vi "SDCP - Read parameter file.vi"(2 "error in (no error)":errorcluster, 3 "Parameter file path":path) -> (0 "error out":errorcluster, 1 "Parameter descriptors":T1[](array[typedef]))   [LabVIEW 2020]
uses:
  Typedefs/SDCP - SMF parameter descriptors.ctl
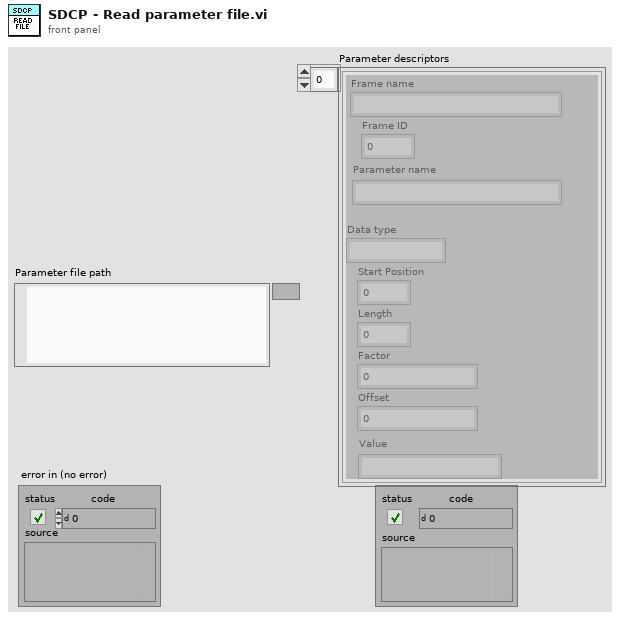
[diagram p1: front panel]
types:
  T1 = typedef "SDCP - SMF parameter descriptors.ctl" = cluster{"Frame name":string, "Frame ID":i32, "Data type":string, "Start Position":i32, "Length":i32, "Factor":dbl, "Offset":dbl, "Parameter name":string, "Value":string}
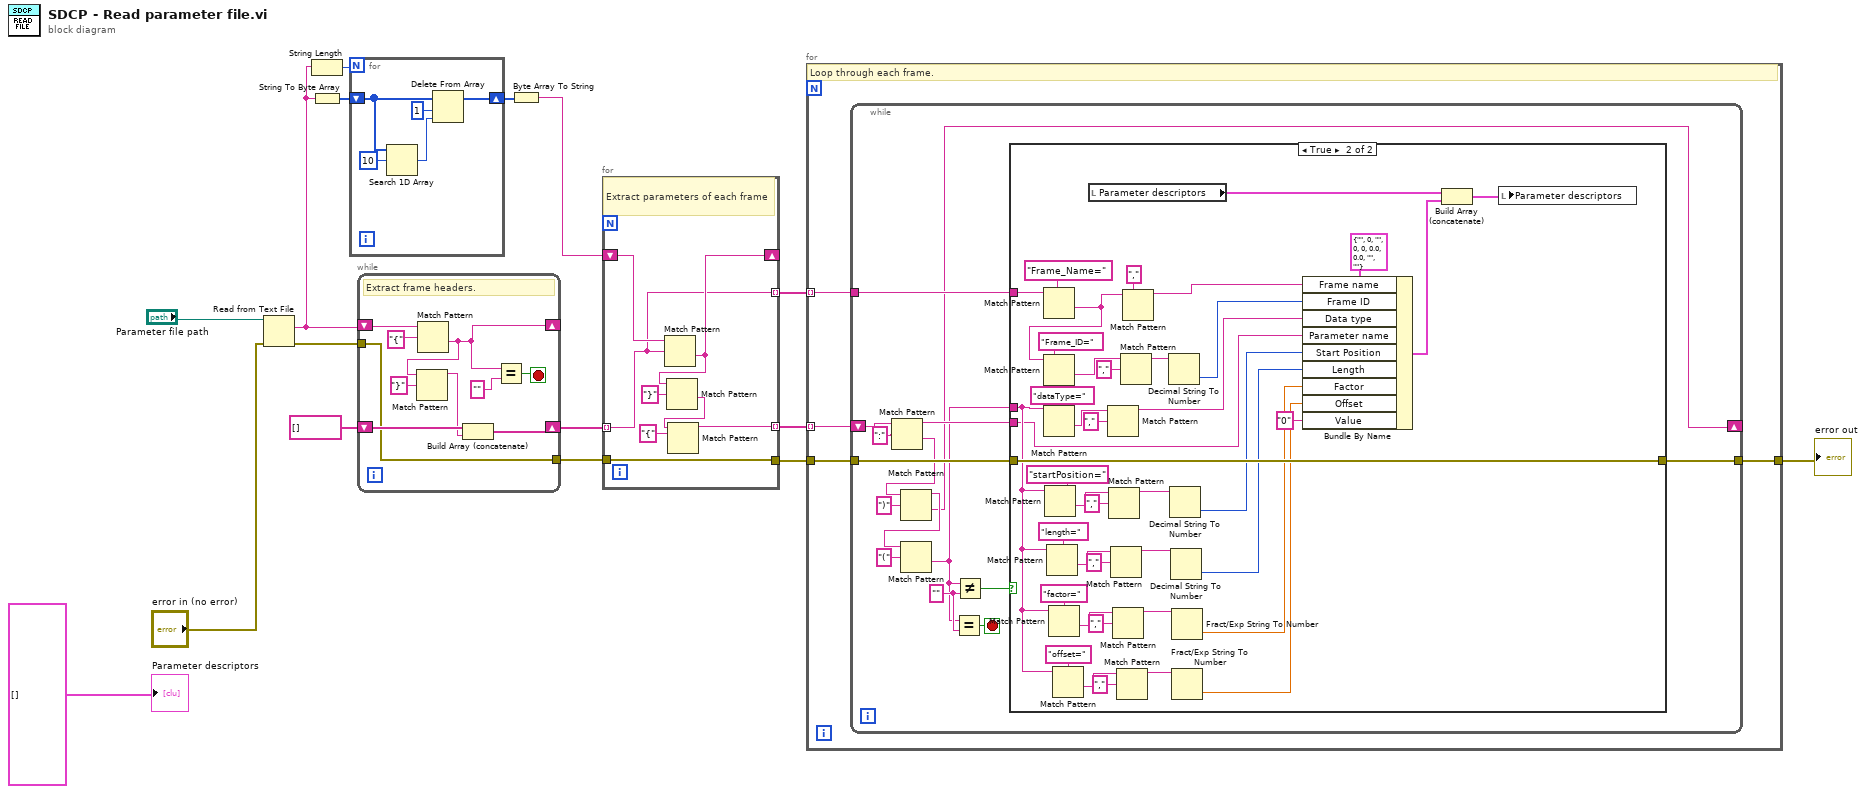
[diagram p0: block diagram]
diagram:
  n1 = Read from Text File(file (use dialog)="Parameter file path", error in="error in (no error)") -> (text=w3:string, error out=w14:errorcluster)  [unwired: 2 in, 2 out]
  n2 = String Length(string=w3) -> (length=w4:i32)
  n3 = String To Byte Array(string=w3) -> (unsigned byte array=w7:u8[])
  n4 = for {
    N: w4 -> [_]
    shift-right: [w21] -> w6
    shift-left: w7 -> [w20]
    n5 = Search 1D Array(1D array=w20, element=u8 10) -> (index of element=w17:i32)  [unwired: 1 in]
    n6 = Delete From Array(array=w20, length=1, index=w17) -> (array with subset deleted=w21:u8[])  [unwired: 1 out]
  }
  n7 = while {
    tunnel: w14 -> [w22]
    shift-right: [w25] -> _
    shift-left: w3 -> [w31]
    shift-right: [w26] -> w12
    shift-left: string[] [] -> [w28]
    tunnel: [w22] -> w11
    stop <- w24 stop-if-true
    # "Extract frame headers."
    n8 = Match Pattern(string=w31, regular expression="{") -> (after substring=w25:string)  [unwired: 1 in, 3 out]
    n9 = Match Pattern(string=w25, regular expression="}") -> (before substring=w27:string)  [unwired: 1 in, 3 out]
    n10 = Build Array (concatenate)(w28, w27) -> (w26:string[])
    n11 = Equal?(x=w25, y="") -> (x = y?=w24:bool)
  }
  n12 = Byte Array To String(unsigned byte array=w6) -> (string=w5:string)
  n13 = for {
    tunnel: w12 -> [w33] mode=indexing
    tunnel: w11 -> [w32]
    shift-right: [w35] -> _
    shift-left: w5 -> [w39]
    tunnel: [w34] -> w9 mode=indexing
    tunnel: [w33] -> w8 mode=indexing
    tunnel: [w32] -> w10
    # "Extract parameters of each frame"
    n14 = Match Pattern(string=w39, regular expression=w33) -> (after substring=w35:string)  [unwired: 1 in, 3 out]
    n15 = Match Pattern(string=w35, regular expression="}") -> (after substring=w38:string)  [unwired: 1 in, 3 out]
    n16 = Match Pattern(string=w38, regular expression="{") -> (before substring=w34:string)  [unwired: 1 in, 3 out]
  }
  n17 = for {
    tunnel: w10 -> [w41]
    tunnel: w9 -> [w42] mode=indexing
    tunnel: w8 -> [w43] mode=indexing
    tunnel: [w40] -> w1
    # "Loop through each frame."
    n18 = while {
      tunnel: w43 -> [w50]
      tunnel: w41 -> [w52]
      tunnel: [w51] -> w40
      shift-right: [w44] -> _
      shift-left: w42 -> [w49]
      stop <- w53 stop-if-true
      w54 = "" ("y")
      n19 = Match Pattern(string=w49, regular expression=":") -> (before substring=w46:string, after substring=w47:string)  [unwired: 1 in, 2 out]
      n20 = Match Pattern(string=w47, regular expression=")") -> (before substring=w57:string, after substring=w44:string)  [unwired: 1 in, 2 out]
      n21 = Match Pattern(string=w57, regular expression="(") -> (after substring=w45:string)  [unwired: 1 in, 3 out]
      n22 = Equal?(x=w45, y=w54) -> (x = y?=w53:bool)
      n23 = Not Equal?(x=w45, y=w54) -> (x != y?=w55:bool)
      n24 = case shown="True" w55 {
        tunnel: w52 -> [w59 w101]
        tunnel: [w59 w101] -> w51
        tunnel: w50 -> [_ w100]
        tunnel: w46 -> [_ w68]
        tunnel: w45 -> [_ w80]
        frame False {
        }
        frame True {
          n25 = Match Pattern(string=w100, regular expression="Frame_Name=") -> (after substring=w97:string)  [unwired: 1 in, 3 out]
          n26 = Match Pattern(string=w97, regular expression="Frame_ID=") -> (after substring=w75:string)  [unwired: 1 in, 3 out]
          n27 = Match Pattern(string=w80, regular expression="dataType=") -> (after substring=w94:string)  [unwired: 1 in, 3 out]
          n28 = Match Pattern(string=w80, regular expression="startPosition=") -> (after substring=w91:string)  [unwired: 1 in, 3 out]
          n29 = Match Pattern(string=w80, regular expression="length=") -> (after substring=w88:string)  [unwired: 1 in, 3 out]
          n30 = Match Pattern(string=w80, regular expression="factor=") -> (after substring=w85:string)  [unwired: 1 in, 3 out]
          n31 = Match Pattern(string=w80, regular expression="offset=") -> (after substring=w82:string)  [unwired: 1 in, 3 out]
          n32 = local read "Parameter descriptors"() -> (w63:T1[])
          n33 = Match Pattern(string=w94, regular expression=",") -> (before substring=w69:string)  [unwired: 1 in, 3 out]
          n34 = Match Pattern(string=w91, regular expression=",") -> (before substring=w76:string)  [unwired: 1 in, 3 out]
          n35 = Match Pattern(string=w88, regular expression=",") -> (before substring=w77:string)  [unwired: 1 in, 3 out]
          n36 = Match Pattern(string=w85, regular expression=",") -> (before substring=w79:string)  [unwired: 1 in, 3 out]
          n37 = Match Pattern(string=w82, regular expression=",") -> (before substring=w78:string)  [unwired: 1 in, 3 out]
          n38 = Match Pattern(string=w75, regular expression=",") -> (before substring=w73:string)  [unwired: 1 in, 3 out]
          n39 = Match Pattern(string=w97, regular expression=",") -> (before substring=w71:string)  [unwired: 1 in, 3 out]
          n40 = Decimal String To Number(string=w73) -> (number=w70:i32)  [unwired: 2 in, 1 out]
          n41 = Decimal String To Number(string=w76) -> (number=w67:i32)  [unwired: 2 in, 1 out]
          n42 = Decimal String To Number(string=w77) -> (number=w66:i32)  [unwired: 2 in, 1 out]
          n43 = Fract/Exp String To Number(string=w79) -> (number=w65:dbl)  [unwired: 3 in, 1 out]
          n44 = Fract/Exp String To Number(string=w78) -> (number=w64:dbl)  [unwired: 3 in, 1 out]
          n45 = Bundle By Name(cluster=T1 {"Frame name"="", "Frame ID"=0, "Data type"="", "Start Position"=0, "Length"=0, "Factor"=0.0, "Offset"=0.0, "Parameter name"="", "Value"=""}, "Frame name"=w71, "Frame ID"=w70, "Data type"=w69, "Parameter name"=w68, "Start Position"=w67, "Length"=w66, "Factor"=w65, "Offset"=w64, "Value"="0") -> (w62:T1)
          n46 = Build Array (concatenate)(w63, w62) -> (w61:T1[])
          n47 = local write "Parameter descriptors"(w61) -> ()
        }
      }
    }
  }
  "error out" <- w1
  "Parameter descriptors" <- T1[] [] ("Parameter descriptors")
